vi "Interface Terminator.vi"(6 "k (0)":i32, 8 "error in (no error)":errorcluster, 9 "j (0)":i32, 10 "i (0)":i32, 11 "VISA resource name":refnum<visa-resource-name>) -> (0 "error out":errorcluster, 3 "VISA resource name out":refnum<visa-resource-name>, 4 "Device Errors":cluster{"code":i32, "Text":string}[](array[cluster]))   [LabVIEW 2014, in "Stanford Research DG645 - Driver.lvlib"]
doc: "Interface Command:XTRM i,j,k\nInstrument Error Check\n\nSet the interface terminator that is appended to each response to i, j, k. The default terminator is 13, 10."
uses:
  Stanford Research DG645 - Driver.lvlib
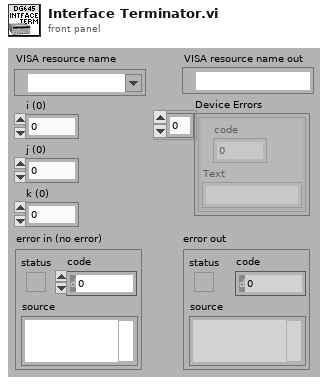
[diagram p1: front panel]
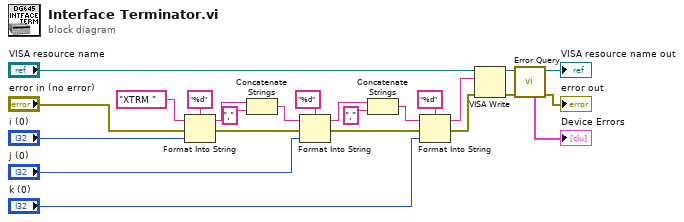
[diagram p0: block diagram]
diagram:
  n1 = Format Into String(format string="%d", initial string="XTRM " ("command"), error in="error in (no error)", "i (0)") -> (resulting string=w8:string, error out=w11:errorcluster)
  n2 = Concatenate Strings(w8, "," ("string")) -> (w6:string)
  n3 = Format Into String(format string="%d", initial string=w6, error in=w11, "j (0)") -> (resulting string=w2:string, error out=w12:errorcluster)
  n4 = Concatenate Strings(w2, "," ("string")) -> (w1:string)
  n5 = Format Into String(format string="%d", initial string=w1, error in=w12, "k (0)") -> (resulting string=w9:string, error out=w10:errorcluster)
  n6 = VISA Write(VISA resource name="VISA resource name", write buffer=w9, error in (no error)=w10) -> (VISA resource name out=w20:refnum<visa-resource-name>, error out=w17:errorcluster)  [unwired: 1 out]
  n7 = call "Error Query.vi"("error in (no error)"=w17, "VISA resource name"=w20) -> ("error out"=→"error out":errorcluster, "VISA resource name out"=→"VISA resource name out":refnum<visa-resource-name>, "Device Errors"=→"Device Errors":cluster{"code":i32, "Text":string}[])  [unwired: 7 in]
